vi "Create Popup Image Window Events.vi"(8 "error in (no error)":errorcluster) -> (0 "error out":errorcluster, 3 "Popup Image Window Events":T1)   [LabVIEW 2020, in "AR Example.lvlib" / "UI.lvclass"]
uses:
  UI.lvclass
  UI.lvclass/UI.ctl
  Popup Image Window Action.ctl
  Popup Image Window Events.ctl
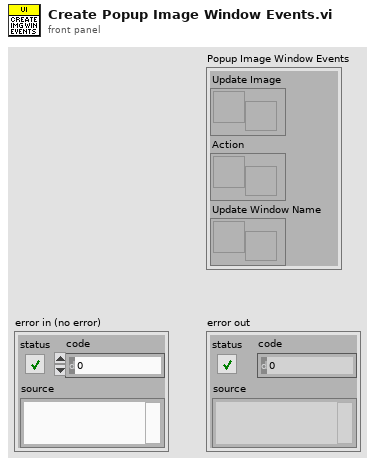
[diagram p1: front panel]
types:
  T1 = typedef "AR Example.lvlib/UI.lvclass/Popup Image Window Events.ctl" = cluster{"Update Image":refnum<user-event>, "Action":refnum<user-event>, "Update Window Name":refnum<user-event>}
  T2 = typedef "AR Example.lvlib/UI.lvclass/Popup Image Window Action.ctl" = enum16{"Show Panel", "Hide Panel", "Exit"}
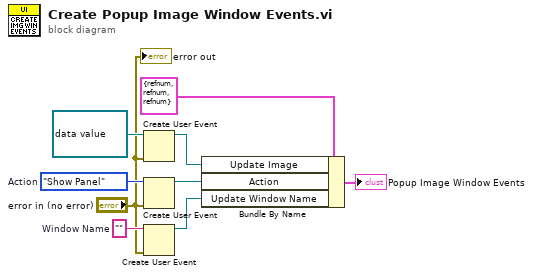
[diagram p0: block diagram]
diagram:
  w3 = ""  # Window Name
  w4 = Popup_Image_Window_Action."Show Panel"  # Action
  n1 = Create User Event(user event datatype=refnum<data-value> refnum ("Image Source"), error in="error in (no error)") -> (user event=w7:refnum<user-event>)  [unwired: 1 out]
  n2 = Create User Event(user event datatype=w4, error in="error in (no error)") -> (user event=w8:refnum<user-event>)  [unwired: 1 out]
  n3 = Create User Event(user event datatype=w3, error in="error in (no error)") -> (user event=w2:refnum<user-event>)  [unwired: 1 out]
  n4 = Bundle By Name(cluster=T1 {"Update Image"=refnum, "Action"=refnum, "Update Window Name"=refnum} ("Popup Image Window Events"), "Update Image"=w7, "Action"=w8, "Update Window Name"=w2) -> (→"Popup Image Window Events":T1)
  "error out" <- "error in (no error)"
